vi "GetVIByName.vi"(8 "error in (no error)":errorcluster, 10 "VI Name":string[](array[string]), 11 "Application in":refnum<class "Application.lvclass">) -> (0 "error out":errorcluster, 2 "VI Reference":refnum<vi>, 3 "Application out":refnum<class "Application.lvclass">)   [LabVIEW 2016, in "Application.lvclass"]
uses:
  Application.lvclass
  Application.lvclass/Application.ctl
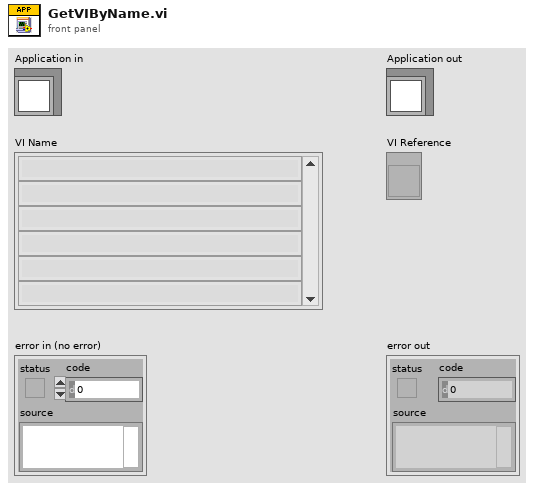
[diagram p1: front panel]
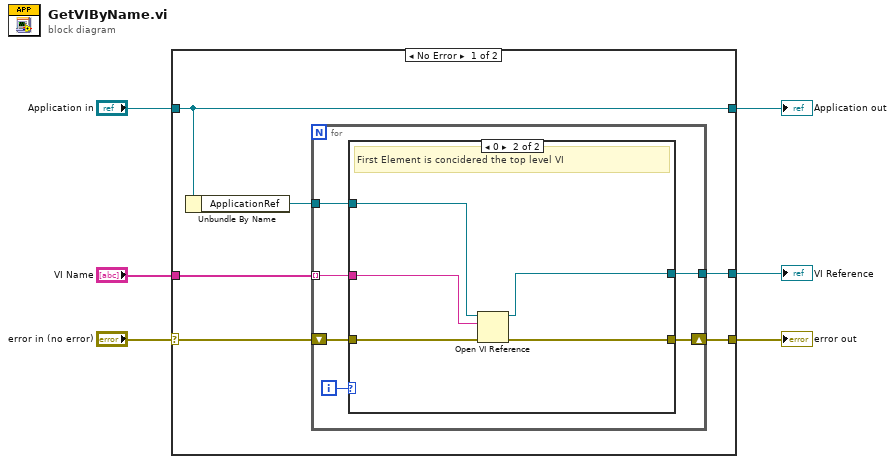
[diagram p0: block diagram]
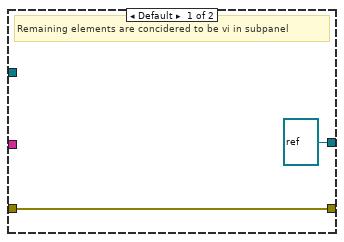
[diagram p2: hidden frame]
diagram:
  n1 = case shown="No Error" "error in (no error)" {
    selector: "error in (no error)" -> [w12 w27]
    tunnel: [w11 w27] -> w5
    tunnel: [w10 w26] -> w3
    tunnel: "Application in" -> [w10 w26]
    tunnel: "VI Name" -> [w8 _]
    tunnel: [w7 _] -> w1
    frame No Error {
      n2 = Unbundle By Name(w10) -> ("ApplicationRef"=w9:refnum<vi>)
      n3 = for {
        tunnel: w9 -> [w16]
        tunnel: w8 -> [w15] mode=indexing
        tunnel: [w14] -> w7
        shift-right: [w17] -> w11
        shift-left: w12 -> [w18]
        i -> [w13]
        n4 = case shown="0" w13 {
          tunnel: w18 -> [w20 w25]
          tunnel: [w20 w24] -> w17
          tunnel: w16 -> [_ w23]
          tunnel: w15 -> [_ w22]
          tunnel: [refnum<vi> refnum ("vi reference") w21] -> w14
          frame Default {
            # "Remaining elements are concidered to be vi in subpanel"
          }
          frame 0 {
            # "First Element is concidered the top level VI"
            n5 = Open VI Reference(application reference (local)=w23, vi path=w22, error in (no error)=w25) -> (vi reference=w21:refnum<vi>, error out=w24:errorcluster)  [unwired: 3 in]
          }
        }
      }
    }
    frame Error {
    }
  }
  "error out" <- w5
  "Application out" <- w3
  "VI Reference" <- w1
